vi "(SubVI) Wang 97 Tether Calibration-Calculate Force and xDNAt.vi"(0 "Xst Array (nm)":dbl[](array[numeric]), 2 "Xbd Array (nm)":dbl[](array[numeric]), 3 "zbd Array (nm)":dbl[](array[numeric]), 5 "Calibration":T1) -> (6 "xDNA":dbl[](array[numeric]), 7 "Force":dbl[](array[numeric]))   [LabVIEW 2014]
uses:
  Calibration.ctl
panel:
  out "Fx":dbl
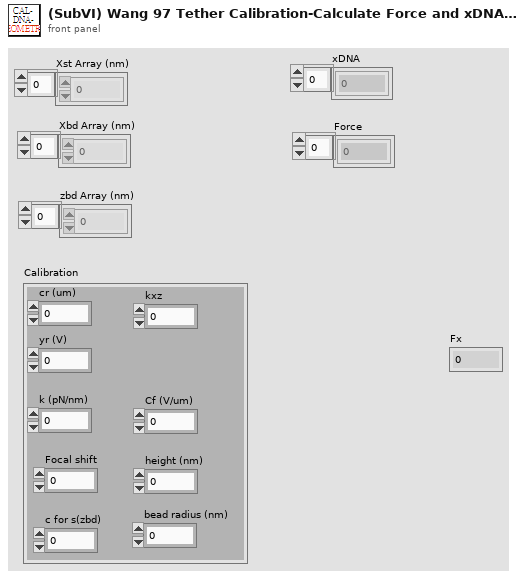
[diagram p1: front panel]
types:
  T1 = typedef "Calibration.ctl" = cluster{"cr (um)":dbl, "yr (V)":dbl, "height (nm)":dbl, "Cf (V/um)":dbl, "kxz":dbl, "k (pN/nm)":dbl, "Focal shift":dbl, "c for s(zbd)":dbl, "bead radius (nm)":dbl}
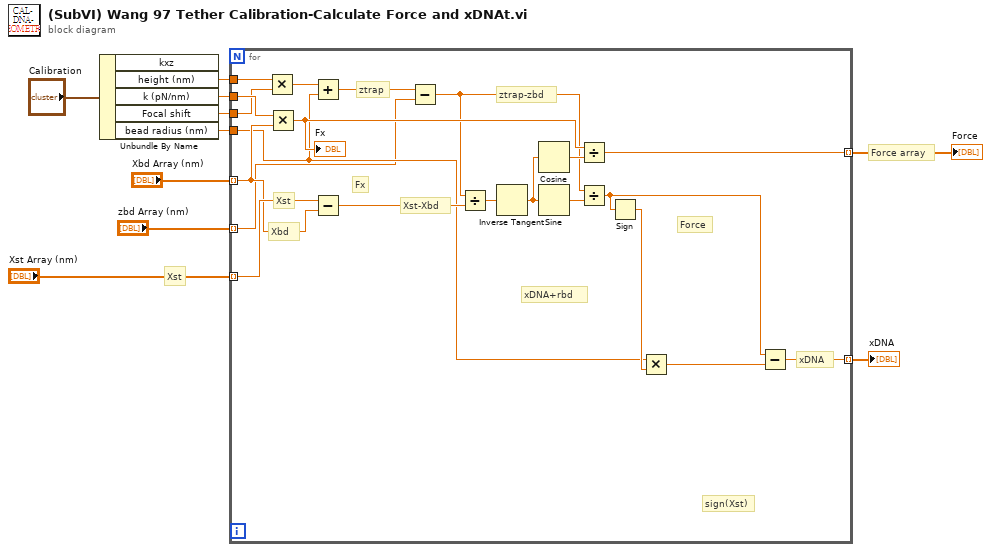
[diagram p0: block diagram]
diagram:
  # "Force array"
  # "Xst"
  n1 = Unbundle By Name("Calibration") -> ("height (nm)"=w3:dbl, "k (pN/nm)"=w5:dbl, "Focal shift"=w4:dbl, "bead radius (nm)"=w2:dbl)  [unwired: 1 out]
  n2 = for {
    tunnel: "Xst Array (nm)" -> [w24] mode=indexing
    tunnel: "Xbd Array (nm)" -> [w20] mode=indexing
    tunnel: [w23] -> w9 mode=indexing
    tunnel: [w22] -> w10 mode=indexing
    tunnel: w5 -> [w15]
    tunnel: w2 -> [w14]
    tunnel: w4 -> [w13]
    tunnel: w3 -> [w12]
    tunnel: "zbd Array (nm)" -> [w11] mode=indexing
    # "ztrap"
    # "xDNA"
    # "xDNA+rbd"
    # "Force"
    # "Fx"
    # "sign(Xst)"
    # "ztrap-zbd"
    # "Xst-Xbd"
    # "Xst"
    # "Xbd"
    n3 = Multiply(x=w12, y=w13) -> (x*y=w16:dbl)
    n4 = Multiply(x=w15, y=w20) -> (x*y=w19:dbl)
    "Fx" <- w19
    n5 = Add(x=w16, y=w14) -> (x+y=w18:dbl)
    n6 = Subtract(x=w24, y=w20) -> (x-y=w31:dbl)
    n7 = Subtract(x=w18, y=w11) -> (x-y=w17:dbl)
    n8 = Divide(x=w17, y=w31) -> (x/y=w30:dbl)
    n9 = Inverse Tangent(1:w30) -> (0:w28:dbl)
    n10 = Cosine(x=w28) -> (cos(x)=w27:dbl)
    n11 = Sine(x=w28) -> (sin(x)=w29:dbl)
    n12 = Divide(x=w19, y=w27) -> (x/y=w22:dbl)
    n13 = Divide(x=w17, y=w29) -> (x/y=w21:dbl)
    n14 = Sign(1:w21) -> (0:w26:dbl)
    n15 = Multiply(x=w14, y=w26) -> (x*y=w25:dbl)
    n16 = Subtract(x=w21, y=w25) -> (x-y=w23:dbl)
  }
  "Force" <- w10
  "xDNA" <- w9
